vi "Read List.vi"(8 "error in (no error)":errorcluster, 11 "StringList Reference":refnum<data-value>) -> (0 "error out":errorcluster, 2 "Items":string[](array[string]), 3 "StringList Reference":refnum<data-value>)   [LabVIEW 2015, in "StringList.lvlib" / "StringList.lvclass"]
uses:
  StringList.lvclass
  StringList.lvclass/StringList.ctl
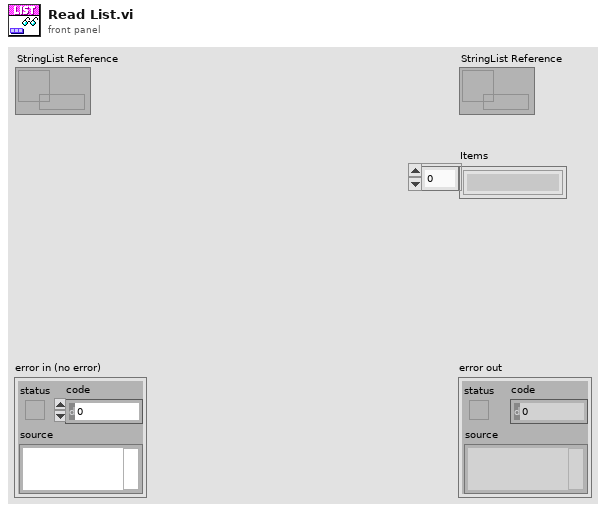
[diagram p1: front panel]
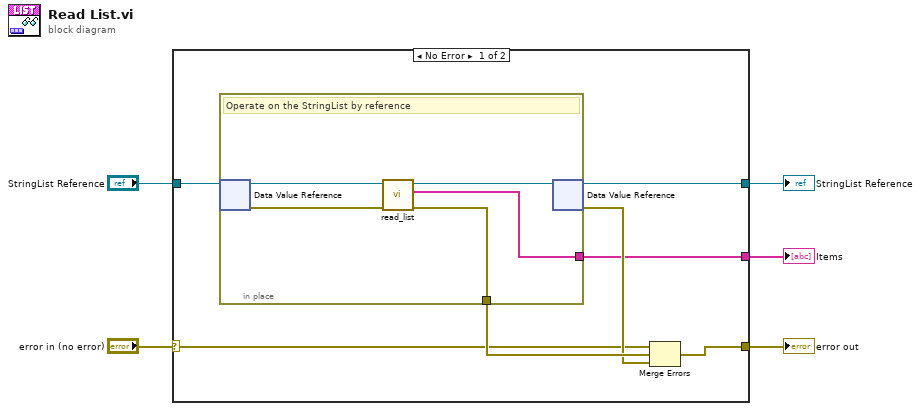
[diagram p0: block diagram]
diagram:
  n1 = case shown="No Error" "error in (no error)" {
    selector: "error in (no error)" -> [w7 w19]
    tunnel: [w12 w19] -> w5
    tunnel: "StringList Reference" -> [w11 w18]
    tunnel: [w10 w18] -> w3
    tunnel: [w6 _] -> w1
    frame No Error {
      n2 = in-place {
        in-place-border: [w14] -> w9
        in-place-border: [w13] -> w6
        # "Operate on the StringList by reference"
        n3 = in-place-dvr #1(w11) -> (w17:refnum<class "StringList.lvclass">, w15:errorcluster)
        n4 = call "read_list.vi"("error in (no error)"=w15, "StringList in"=w17) -> ("error out"=w14:errorcluster, "List Items"=w13:string[], "StringList out"=w16:refnum<class "StringList.lvclass">)  [unwired: 7 in]
        n5 = in-place-dvr #1(w16) -> (w10:refnum<data-value>, w8:errorcluster)
      }
      n6 = Merge Errors(w7, w9, w8) -> (w12:errorcluster)
    }
    frame Error {
    }
  }
  "error out" <- w5
  "StringList Reference" <- w3
  "Items" <- w1
